vi "Close kinect systems.vi"(8 "error in (no error)":errorcluster, 10 "Kinect Handle":i64, 11 "Video handle in":i64) -> (0 "error out":errorcluster)   [LabVIEW 2017]
uses:
  subVIs/Led Control.ctl
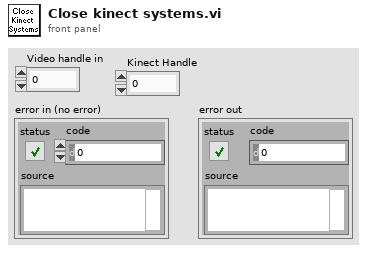
[diagram p1: front panel]
types:
  T1 = typedef "Led Control.ctl" = enum32{"LED_OFF", "LED_GREEN", "LED_RED", "LED_YELLOW", "LED_BLINK_GREEN", "LED_BLINK_GREEN2", "LED_BLINK_RED_YELLOW"}
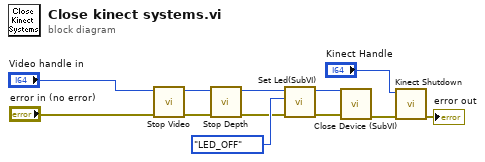
[diagram p0: block diagram]
diagram:
  n1 = call "Stop Video.vi"("error in (no error)"="error in (no error)", "handle in"="Video handle in") -> ("error out"=w9:errorcluster, "handle out"=w8:i64)  [unwired: 7 in, 1 out]
  n2 = call "Stop Depth.vi"("error in (no error)"=w9, "handle in"=w8) -> ("error out"=w6:errorcluster, "handle out"=w7:i64)  [unwired: 7 in, 1 out]
  n3 = call "Set Led(SubVI).vi"("error in (no error)"=w6, "Led Option"=Led_Control."LED_OFF", "handle in"=w7) -> ("error out"=w4:errorcluster, "handle out"=w5:i64)  [unwired: 7 in]
  n4 = call "Close Device (SubVI).vi"("error in (no error)"=w4, "handle in"=w5) -> ("error out"=w2:errorcluster)  [unwired: 8 in, 1 out]
  n5 = call "Kinect Shutdown.vi"("error in (no error)"=w2, "Device_handle"="Kinect Handle") -> ("error out"=→"error out":errorcluster)  [unwired: 9 in]
